vi "Loop_SM.vi"() -> ()   [LabVIEW 2017, in "Wing.lvlib"]
uses:
  Wing.lvlib
  ENUM_SM_Action.ctl
  ENUM_SM_State.ctl
  Global_SM Write_Data Out.vi
  Global_CMD.vi
  System Drivers/Phoenix-LabVIEW/Motor Controller/Controls/CTRE_Phoenix_MotorControl_ControlMode.ctl
  _SHARE ALL/RoboRio Share All/SRX Share All/TypeDefs SRX/Cluster_SRX_Mode and Value.ctl
  _SHARE ALL/RoboRio Share All/SRX Share All/TypeDefs SRX/Cluster_SRX_Analog In Data.ctl
  _SHARE ALL/Global Share All/Global_STOP.vi
  Global_ACT Write_Data Out.vi
  <vilib>/Rock Robotics/WPI/DriverStation/WPI_DriverStationMatch Info.ctl
panel:
  out "Wing_SM_WinchMode":T1 items=["PercentOutput"=0, "Position"=1, "Velocity"=2, "Current"=3, "Follower"=5, "MotionProfile"=6, "MotionMagic"=7, "MotionMagicArc"=8, "MotionProfileArc"=10, "Disabled"=15]
  in  "Match Info":T2={"Autonomous Elapsed Seconds"=0.0, "TeleOp Elapsed Seconds"=0.0, "Disabled Elapsed Seconds"=0.0, "Visited Autonomous"=FALSE, "Visited TeleOp"=FALSE, "Visited Disabled"=FALSE, "Autonomous Settings"={"Autonomous Style"=enum."Independent", "VI Refnum"=refnum}}
  out "Sm Winch DBL Data":dbl
  out "Output Bool Data":bool
  out "Cycle Time (S)":dbl format="%.3g"
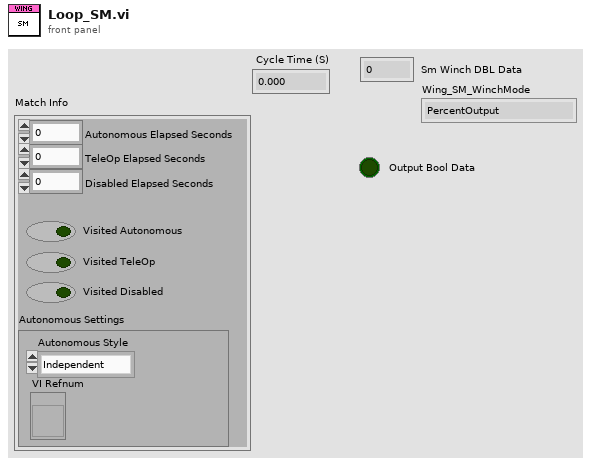
[diagram p1: front panel]
types:
  T1 = typedef "CTRE_Phoenix_MotorControl_ControlMode.ctl" = u16
  T2 = typedef "WPI_DriverStationMatch Info.ctl" = cluster{"Autonomous Elapsed Seconds":dbl, "TeleOp Elapsed Seconds":dbl, "Disabled Elapsed Seconds":dbl, "Visited Autonomous":bool, "Visited TeleOp":bool, "Visited Disabled":bool, "Autonomous Settings":cluster{"Autonomous Style":enum16{"Iterative", "Independent"}, "VI Refnum":refnum<vi>}}
  T3 = typedef "Cluster_SRX_Analog In Data.ctl" = cluster{"WithOv":i32, "Raw":i32, "Velocity":i32}
  T4 = typedef "Cluster_SRX_Mode and Value.ctl" = cluster{"Mode":T1, "Value":dbl}
  T5 = typedef "Wing.lvlib/ENUM_SM_State.ctl" = enum16{"Startup", "Disabled", "Shutdown", "Closed", "Opening", "Open Lowered", "Open Raising", "Open Raised", "Open Lowering", "Closing"}
  T6 = typedef "Wing.lvlib/ENUM_SM_Action.ctl" = enum16{"No Action", "Piston Open", "Piston Close", "Start Up", "Shut Down", "Raise Winch", "Lower Winch"}
  T7 = cluster{"State":T5, "Previous State":T5, "Current Time":timestamp, "Previous Time":timestamp, "Start Time":timestamp, "Target Time (ms)":u32, "Cycle Time(S)":dbl, "Wing_SM Winch Value":dbl, "SM Input DBL":dbl, "Wing_SM_WinchMode":T1, "SM Solen Bool":bool, "Mode And Value":T4, "Analog Sensor Data Out":T3, "Match Info":T2, "Test Mode?":bool, "Lower Bool":bool, "Raise Bool":bool}
  T8 = typedef "Cluster_SRX_Common Runtime Data.ctl" = cluster{"Calc":T9, "Voltage ":T10, "Sensor":T11, "Current":dbl, "Temp":dbl}
  T9 = typedef "Cluster_SRX_Error Calculations.ctl" = cluster{"Error":i32, "D-Error":dbl, "I-Acc":dbl}
  T10 = typedef "Cluster_SRX_Voltage Out Data.ctl" = cluster{"Percent":dbl, "Output":dbl, "Bus":dbl}
  T11 = typedef "Cluster_SRX_Sensor Out Data.ctl" = cluster{"Pos":i32, "Vel":i32}
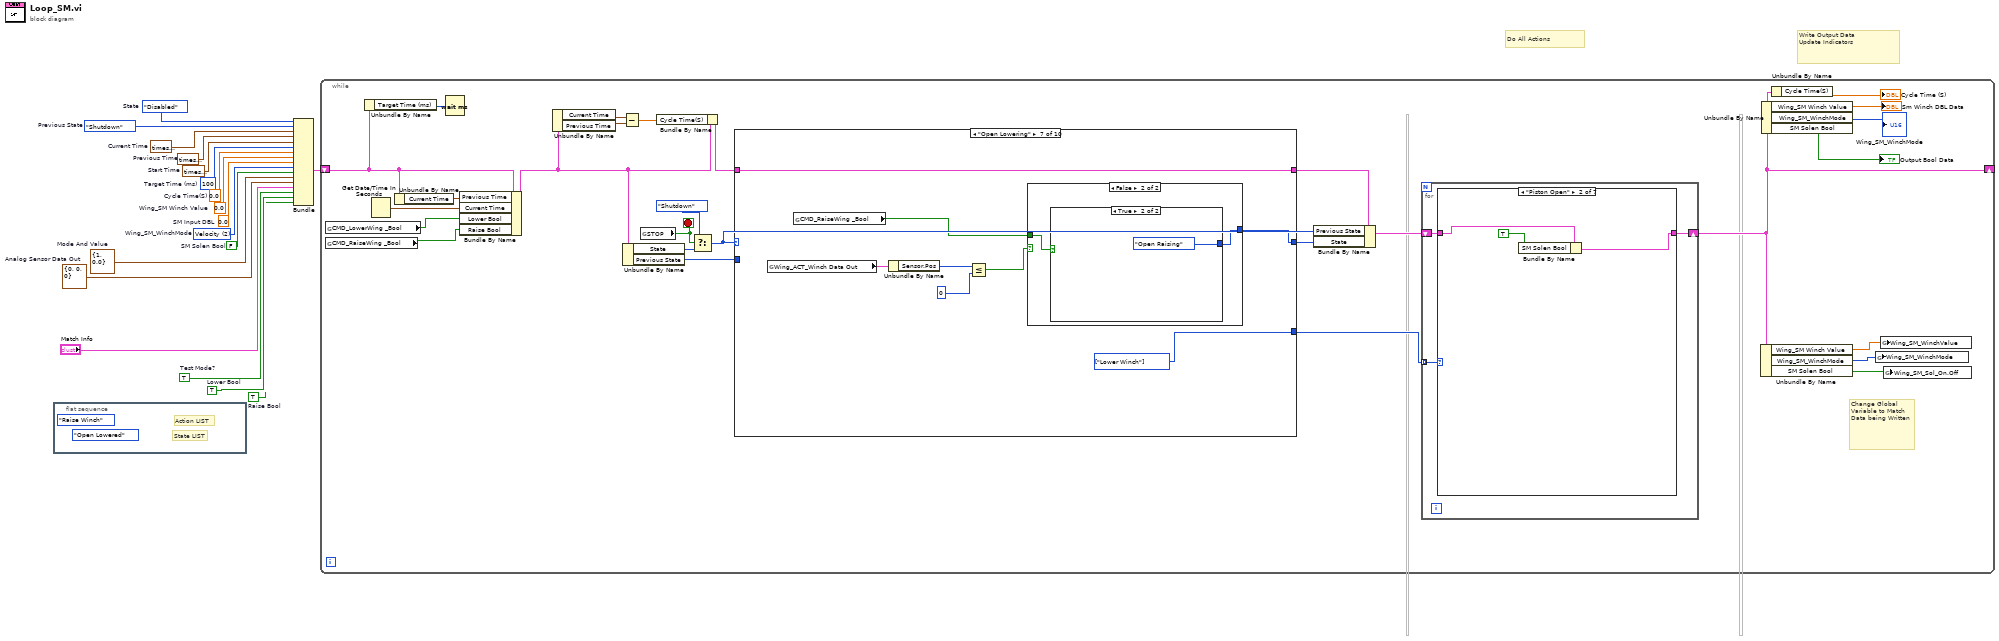
[diagram p0: block diagram]
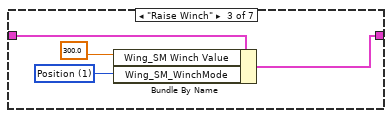
[diagram p3: hidden frame]
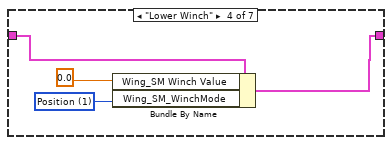
[diagram p4: hidden frame]
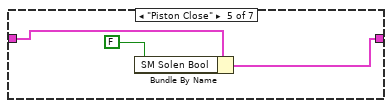
[diagram p5: hidden frame]
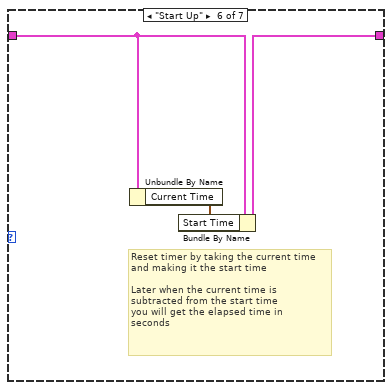
[diagram p6: hidden frame]
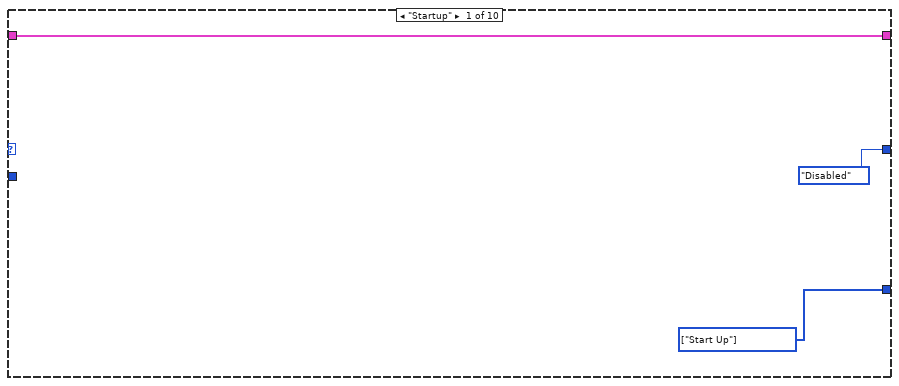
[diagram p8: hidden frame]
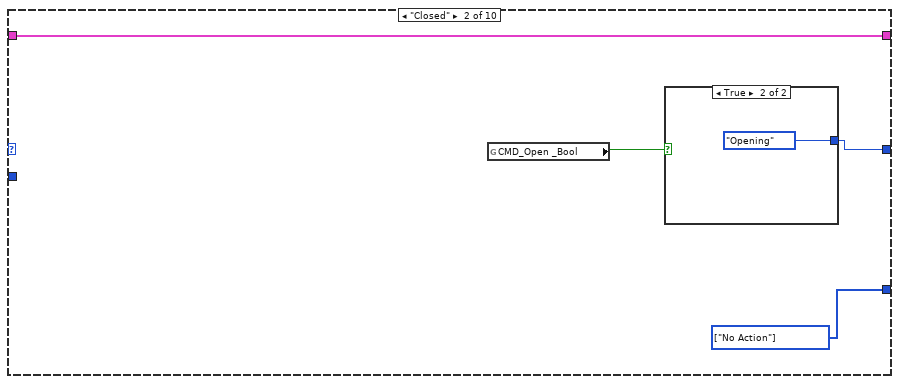
[diagram p9: hidden frame]
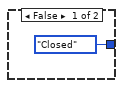
[diagram p10: hidden frame]
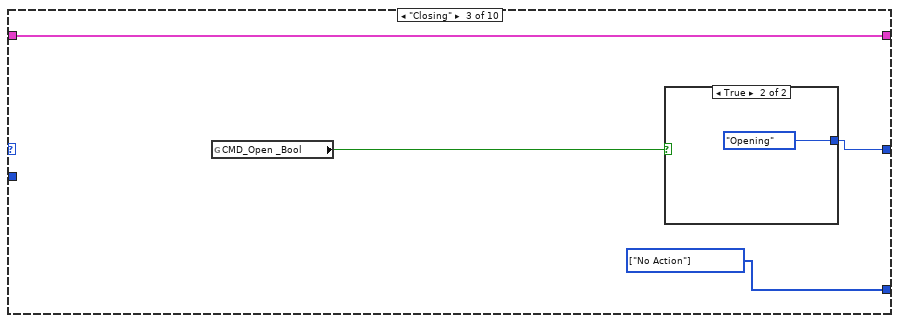
[diagram p11: hidden frame]
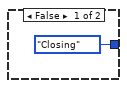
[diagram p12: hidden frame]
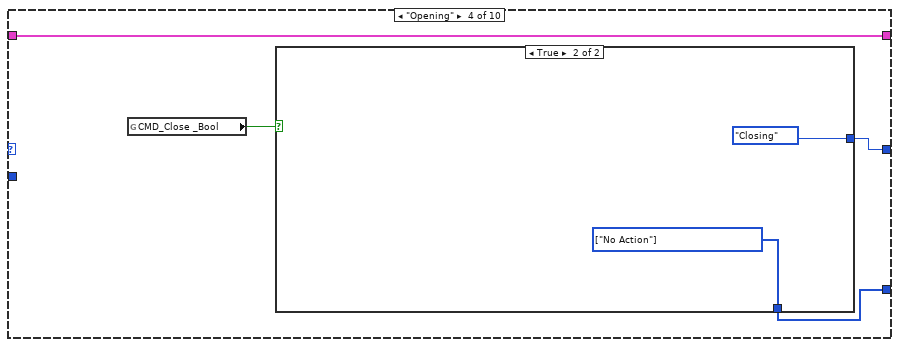
[diagram p13: hidden frame]
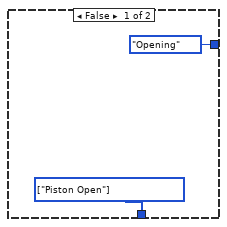
[diagram p14: hidden frame]
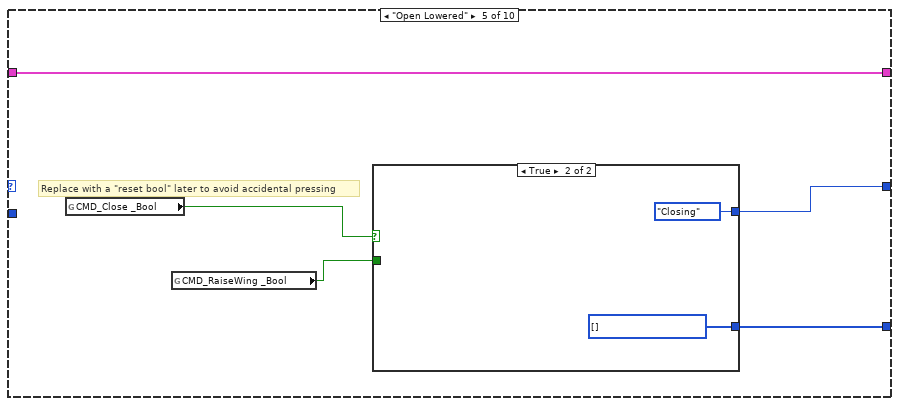
[diagram p15: hidden frame]
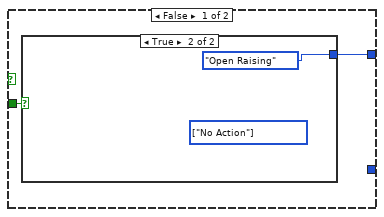
[diagram p16: hidden frame]
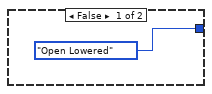
[diagram p17: hidden frame]
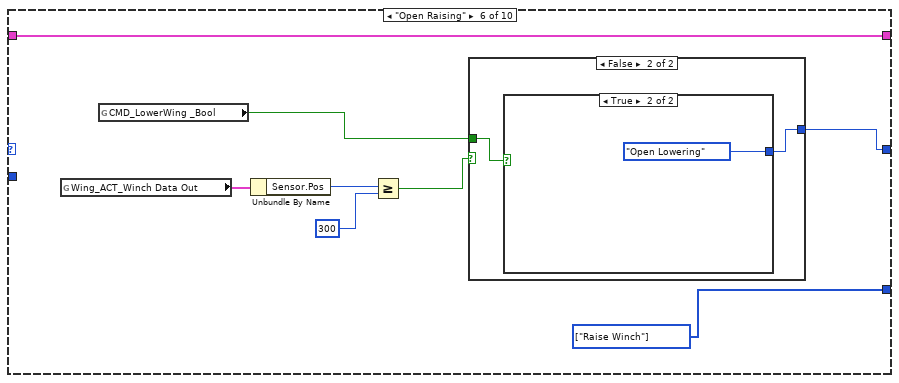
[diagram p18: hidden frame]
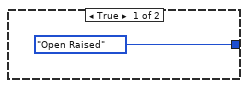
[diagram p19: hidden frame]
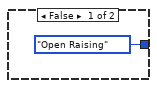
[diagram p20: hidden frame]
diagram:
  w1 = T1 2 items=["PercentOutput"=0, "Position"=1, "Velocity"=2, "Current"=3, "Follower"=5, "MotionProfile"=6, "MotionMagic"=7, "MotionMagicArc"=8, "MotionProfileArc"=10, "Disabled"=15]  # Wing_SM_WinchMode
  w2 = TRUE  # Raise Bool
  w3 = TRUE  # Lower Bool
  w4 = TRUE  # Test Mode?
  w6 = T3 {"WithOv"=0, "Raw"=0, "Velocity"=0}  # Analog Sensor Data Out
  w7 = T4 {"Mode"=1, "Value"=0.0}  # Mode And Value
  w8 = 0.0  # Cycle Time(S)
  w9 = ENUM_SM_State."Shutdown"  # Previous State
  w10 = timestamp(0 s since 1904-01-01)  # Previous Time
  w11 = FALSE  # SM Solen Bool
  w12 = u32 100  # Target Time (ms)
  w13 = 0.0  # SM Input DBL
  w14 = 0.0  # Wing_SM Winch Value
  w15 = timestamp(0 s since 1904-01-01)  # Start Time
  w16 = timestamp(0 s since 1904-01-01)  # Current Time
  w17 = ENUM_SM_State."Disabled"  # State
  # "Do All Actions"
  # "Write Output Data\nUpdate Indicators"
  n1 = flat-sequence {
    frame #0 {
      (unwired) ENUM_SM_State."Open Lowered" ("State")
      (unwired) ENUM_SM_Action."Raise Winch" ("Action")
      # "State LIST"
      # "Action LIST"
    }
  }
  n2 = Bundle("State"=w17, "Previous State"=w9, "Current Time"=w16, "Previous Time"=w10, "Start Time"=w15, "Target Time (ms)"=w12, "Cycle Time(S)"=w8, "Wing_SM Winch Value"=w14, "SM Input DBL"=w13, "Wing_SM_WinchMode"=w1, "SM Solen Bool"=w11, "Mode And Value"=w7, "Analog Sensor Data Out"=w6, "Match Info"="Match Info", "Test Mode?"=w4, "Lower Bool"=w3, "Raise Bool"=w2) -> (w18:T7)  [unwired: 1 in]
  n3 = while {
    shift-right: [w35] -> _
    shift-left: w18 -> [w38]
    stop <- w43 stop-if-true
    # "Change Global\nVariable to Match\nData being Written"
    n4 = global read "Global_CMD.vi" "CMD_LowerWing _Bool"() -> (w26:bool)
    n5 = global read "Global_CMD.vi" "CMD_RaiseWing _Bool"() -> (w25:bool)
    n6 = Unbundle By Name(w38) -> ("Target Time (ms)"=w40:u32)
    n7 = Get Date/Time In Seconds() -> (seconds since 1Jan1904=w46:timestamp)
    n8 = Unbundle By Name(w38) -> ("Current Time"=w39:timestamp)
    n9 = Wait (ms)(milliseconds to wait=w40) -> ()  [unwired: 1 out]
    n10 = Bundle By Name(cluster=w38, "Previous Time"=w39, "Current Time"=w46, "Lower Bool"=w26, "Raise Bool"=w25) -> (w31:T7)
    n11 = Unbundle By Name(w31) -> ("Current Time"=w32:timestamp, "Previous Time"=w33:timestamp)
    n12 = Subtract(x=w32, y=w33) -> (x-y=w29:dbl)
    n13 = Unbundle By Name(w31) -> ("State"=w41:T5, "Previous State"=w37:T5)
    n14 = global read "Global_STOP.vi" "STOP"() -> (w43:bool)
    n15 = Bundle By Name(cluster=w31, "Cycle Time(S)"=w29) -> (w30:T7)
    n16 = Select(t=ENUM_SM_State."Shutdown" ("State"), s=w43, f=w41) -> (s? t:f=w21:T5)
    n17 = case shown="\"Open Lowering\"" w21 {
      tunnel: w30 -> [w71 w75 w81 w86 w96 w110 w123 w132 w140 w150]
      tunnel: [w71 w75 w81 w86 w96 w110 w123 w132 w140 w150] -> w44
      tunnel: w37 -> [_ _ _ _ _ _ _ _ _ _]
      tunnel: [ENUM_SM_State."Disabled" ("State") w73 w79 w85 w94 w108 w121 w130 w136 ENUM_SM_State."Shutdown" ("State")] -> w27
      tunnel: [w69 w72 w78 w84 w92 w103 w116 w129 w135 w148] -> w19
      frame "Startup" {
        w69 = T6[] [enum."Start Up"] items=["No Action", "Piston Open", "Piston Close", "Start Up", "Shut Down", "Raise Winch", "Lower Winch"] ("Actions")
      }
      frame "Closed" {
        w72 = T6[] [enum."No Action"] items=["No Action", "Piston Open", "Piston Close", "Start Up", "Shut Down", "Raise Winch", "Lower Winch"] ("Actions")
        n18 = global read "Global_CMD.vi" "CMD_Open _Bool"() -> (w74:bool)
        n19 = case shown="True" w74 {
          tunnel: [ENUM_SM_State."Closed" ("State") ENUM_SM_State."Opening" ("State")] -> w73
          frame False {
          }
          frame True {
          }
        }
      }
      frame "Closing" {
        w78 = T6[] [enum."No Action"] items=["No Action", "Piston Open", "Piston Close", "Start Up", "Shut Down", "Raise Winch", "Lower Winch"] ("Actions")
        n20 = global read "Global_CMD.vi" "CMD_Open _Bool"() -> (w80:bool)
        n21 = case shown="True" w80 {
          tunnel: [ENUM_SM_State."Closing" ("State") ENUM_SM_State."Opening" ("State")] -> w79
          frame False {
          }
          frame True {
          }
        }
      }
      frame "Opening" {
        n22 = global read "Global_CMD.vi" "CMD_Close _Bool"() -> (w87:bool)
        n23 = case shown="True" w87 {
          tunnel: [ENUM_SM_State."Opening" ("State") ENUM_SM_State."Closing" ("State")] -> w85
          tunnel: [w88 w90] -> w84
          frame False {
            w88 = T6[] [enum."Piston Open"] items=["No Action", "Piston Open", "Piston Close", "Start Up", "Shut Down", "Raise Winch", "Lower Winch"] ("Actions")
          }
          frame True {
            w90 = T6[] [enum."No Action"] items=["No Action", "Piston Open", "Piston Close", "Start Up", "Shut Down", "Raise Winch", "Lower Winch"] ("Actions")
          }
        }
      }
      frame "Open Lowered" {
        # "Replace with a \"reset bool\" later to avoid accidental pressing"
        n24 = global read "Global_CMD.vi" "CMD_Close _Bool"() -> (w95:bool)
        n25 = global read "Global_CMD.vi" "CMD_RaiseWing _Bool"() -> (w93:bool)
        n26 = case shown="True" w95 {
          tunnel: [w98 ENUM_SM_State."Closing" ("State")] -> w94
          tunnel: w93 -> [w97 _]
          tunnel: [_ w101] -> w92
          frame False {
            n27 = case shown="True" w97 {
              tunnel: [ENUM_SM_State."Open Lowered" ("State") ENUM_SM_State."Open Raising" ("State")] -> w98
              frame False {
              }
              frame True {
                (unwired) T6[] [enum."No Action"] items=["No Action", "Piston Open", "Piston Close", "Start Up", "Shut Down", "Raise Winch", "Lower Winch"] ("Actions")
              }
            }
          }
          frame True {
            w101 = T6[] [] items=["No Action", "Piston Open", "Piston Close", "Start Up", "Shut Down", "Raise Winch", "Lower Winch"] ("Actions")
          }
        }
      }
      frame "Open Raising" {
        w103 = T6[] [enum."Raise Winch"] items=["No Action", "Piston Open", "Piston Close", "Start Up", "Shut Down", "Raise Winch", "Lower Winch"] ("Actions")
        n28 = global read "Global_ACT Write_Data Out.vi" "Wing_ACT_Winch Data Out"() -> (w107:T8)
        n29 = global read "Global_CMD.vi" "CMD_LowerWing _Bool"() -> (w109:bool)
        n30 = Unbundle By Name(w107) -> ("Sensor.Pos"=w106:i32)
        n31 = Greater Or Equal?(x=w106, y=300) -> (x >= y?=w104:bool)
        n32 = case shown="False" w104 {
          tunnel: w109 -> [_ w113]
          tunnel: [ENUM_SM_State."Open Raised" ("State") w112] -> w108
          frame True {
          }
          frame False {
            n33 = case shown="True" w113 {
              tunnel: [ENUM_SM_State."Open Raising" ("State") ENUM_SM_State."Open Lowering" ("State")] -> w112
              frame False {
              }
              frame True {
              }
            }
          }
        }
      }
      frame "Open Lowering" {
        w116 = T6[] [enum."Lower Winch"] items=["No Action", "Piston Open", "Piston Close", "Start Up", "Shut Down", "Raise Winch", "Lower Winch"] ("Actions")
        n34 = global read "Global_ACT Write_Data Out.vi" "Wing_ACT_Winch Data Out"() -> (w120:T8)
        n35 = global read "Global_CMD.vi" "CMD_RaiseWing _Bool"() -> (w122:bool)
        n36 = Unbundle By Name(w120) -> ("Sensor.Pos"=w119:i32)
        n37 = Less Or Equal?(x=w119, y=0) -> (x <= y?=w117:bool)
        n38 = case shown="False" w117 {
          tunnel: w122 -> [_ w126]
          tunnel: [ENUM_SM_State."Open Lowered" ("State") w125] -> w121
          frame True {
          }
          frame False {
            n39 = case shown="True" w126 {
              tunnel: [ENUM_SM_State."Open Lowering" ("State") ENUM_SM_State."Open Raising" ("State")] -> w125
              frame False {
              }
              frame True {
              }
            }
          }
        }
      }
      frame "Open Raised" {
        w129 = T6[] [enum."No Action"] items=["No Action", "Piston Open", "Piston Close", "Start Up", "Shut Down", "Raise Winch", "Lower Winch"] ("Actions")
        n40 = global read "Global_CMD.vi" "CMD_LowerWing _Bool"() -> (w131:bool)
        n41 = case shown="False" w131 {
          tunnel: [ENUM_SM_State."Open Raised" ("State") ENUM_SM_State."Open Lowering" ("State")] -> w130
          frame False {
          }
          frame True {
          }
        }
      }
      frame "Disabled" {
        w135 = T6[] [enum."No Action"] items=["No Action", "Piston Open", "Piston Close", "Start Up", "Shut Down", "Raise Winch", "Lower Winch"] ("Actions")
        n42 = Unbundle By Name(w140) -> ("Test Mode?"=w139:bool)
        n43 = Unbundle By Name(w140) -> ("Match Info.Autonomous Elapsed Seconds"=w145:dbl, "Match Info.TeleOp Elapsed Seconds"=w144:dbl)
        n44 = Not(x=w139) -> (.not. x?=w138:bool)
        n45 = Add(x=w145, y=w144) -> (x+y=w143:dbl)
        n46 = Less?(x=w143, y=150.0) -> (x < y?=w141:bool)
        n47 = And(x=w141, y=w138) -> (x .and. y?=w137:bool)
        n48 = case shown="False" w137 {
          tunnel: [ENUM_SM_State."Closed" ("State") ENUM_SM_State."Disabled" ("State")] -> w136
          frame False {
          }
          frame True {
          }
        }
      }
      frame "Shutdown" {
        w148 = T6[] [enum."Shut Down"] items=["No Action", "Piston Open", "Piston Close", "Start Up", "Shut Down", "Raise Winch", "Lower Winch"] ("Actions")
      }
    }
    n49 = Bundle By Name(cluster=w44, "Previous State"=w21, "State"=w27) -> (w45:T7)
    n50 = for {
      tunnel: w19 -> [w49] mode=indexing
      shift-right: [w48] -> w35
      shift-left: w45 -> [w47]
      n51 = case shown="\"Piston Open\"" w49 {
        tunnel: w47 -> [w50 w53 w57 w61 w63 w67 w68]
        tunnel: [w50 w51 w56 w60 w62 w66 w68] -> w48
        frame "No Action" {
        }
        frame "Piston Open" {
          n52 = Bundle By Name(cluster=w53, "SM Solen Bool"=TRUE) -> (w51:T7)
        }
        frame "Raise Winch" {
          w55 = T1 1 items=["PercentOutput"=0, "Position"=1, "Velocity"=2, "Current"=3, "Follower"=5, "MotionProfile"=6, "MotionMagic"=7, "MotionMagicArc"=8, "MotionProfileArc"=10, "Disabled"=15] ("Wing_SM_WinchMode")
          n53 = Bundle By Name(cluster=w57, "Wing_SM Winch Value"=300.0, "Wing_SM_WinchMode"=w55) -> (w56:T7)
        }
        frame "Lower Winch" {
          w59 = T1 1 items=["PercentOutput"=0, "Position"=1, "Velocity"=2, "Current"=3, "Follower"=5, "MotionProfile"=6, "MotionMagic"=7, "MotionMagicArc"=8, "MotionProfileArc"=10, "Disabled"=15] ("Wing_SM_WinchMode")
          n54 = Bundle By Name(cluster=w61, "Wing_SM Winch Value"=0.0, "Wing_SM_WinchMode"=w59) -> (w60:T7)
        }
        frame "Piston Close" {
          n55 = Bundle By Name(cluster=w63, "SM Solen Bool"=FALSE) -> (w62:T7)
        }
        frame "Start Up" {
          # "Reset timer by taking the current time\nand making it the start time\n\nLater when the current time is \nsubtracted from the start time\nyou will get the elapsed time in \nseconds"
          n56 = Unbundle By Name(w67) -> ("Current Time"=w65:timestamp)
          n57 = Bundle By Name(cluster=w67, "Start Time"=w65) -> (w66:T7)
        }
        frame "Shut Down" {
        }
      }
    }
    n58 = Unbundle By Name(w35) -> ("Wing_SM Winch Value"=w24:dbl, "Wing_SM_WinchMode"=w22:T1, "SM Solen Bool"=w23:bool)
    n59 = Unbundle By Name(w35) -> ("Wing_SM Winch Value"=→"Sm Winch DBL Data":dbl, "Wing_SM_WinchMode"=→"Wing_SM_WinchMode":T1, "SM Solen Bool"=→"Output Bool Data":bool)
    n60 = Unbundle By Name(w35) -> ("Cycle Time(S)"=→"Cycle Time (S)":dbl)
    n61 = global write "Global_SM Write_Data Out.vi" "Wing_SM_WinchMode"(w22) -> ()
    n62 = global write "Global_SM Write_Data Out.vi" "Wing_SM_WinchValue"(w24) -> ()
    n63 = global write "Global_SM Write_Data Out.vi" "Wing_SM_Sol_On.Off"(w23) -> ()
  }
